vi "LJstreamM write config.vi"(0 "Working Directory":path, 1 "Data File Prefix":string="data", 2 "Scan Rate (Hz)":dbl=100.0 format="%.3f", 3 "Graph History":i32=1000 min=0, 4 "# Channels":i32=4, 5 "filename":string="LJM_Default_Configs.cfg\nLJM_Default_Configs.cfg", 6 "Disable Scaling":bool, 7 "Max File Size (Bytes)":i32=1048576, 9 "Write To File":bool, 10 "Channel Setup":T1={"+Ch"=["0", "1", "2", "3", "4", "5", "6", "7"], "-Ch"=["199", "199", "199", "199", "199", "199", "199", "199"], "Ranges"=[0, 0, 0, 0, 0, 0, 0, 0], "Scaling Equation"=["y=v0", "y=v1", "y=v2", "y=v3", "y=v4", "y=v5", "y=v6", "y=v7"], "Graph?"=[]} {"Ranges" items=["LJ_rgBIP10V", "LJ_rgBIP5V", "LJ_rgUNI5V", "LJ_rgUNI2P5V", "LJ_rgUNI1P25V", "LJ_rgBIP1V", "LJ_rgUNIP625V", "LJ_rgBIPP1V", "LJ_rgBIPP01V"]}, 11 "App Name":string="LJStreamM.cfg", 12 "Interval (ms)":u32=500, 13 "Resolution":u8, 14 "SettlingFactor":u8) -> (15 "error out":errorcluster={"status"=TRUE, "code"=1, "source"="Open/Create/Replace File in NI_LVConfig.lvlib:Load.vi->NI_LVConfig.lvlib:Open Config Data (compatibility).vi->LJstreamM write config.vi<APPEND>\nLJM_Default_Configs.cfg\nLJM_Default_Configs.cfg:\\"})   [LabVIEW 2025]
uses:
  LJstreamM globals.vi
  <vilib>/Utility/config.llb/Write Key (String).vi
  <vilib>/Utility/config.llb/Write Key (U32).vi
  <vilib>/Utility/config.llb/Write Key (Double).vi
  <vilib>/Utility/config.llb/Write Key (I32).vi
  <vilib>/Utility/config.llb/Write Key (Boolean).vi
  <vilib>/Utility/config.llb/NI_LVConfig.lvlib
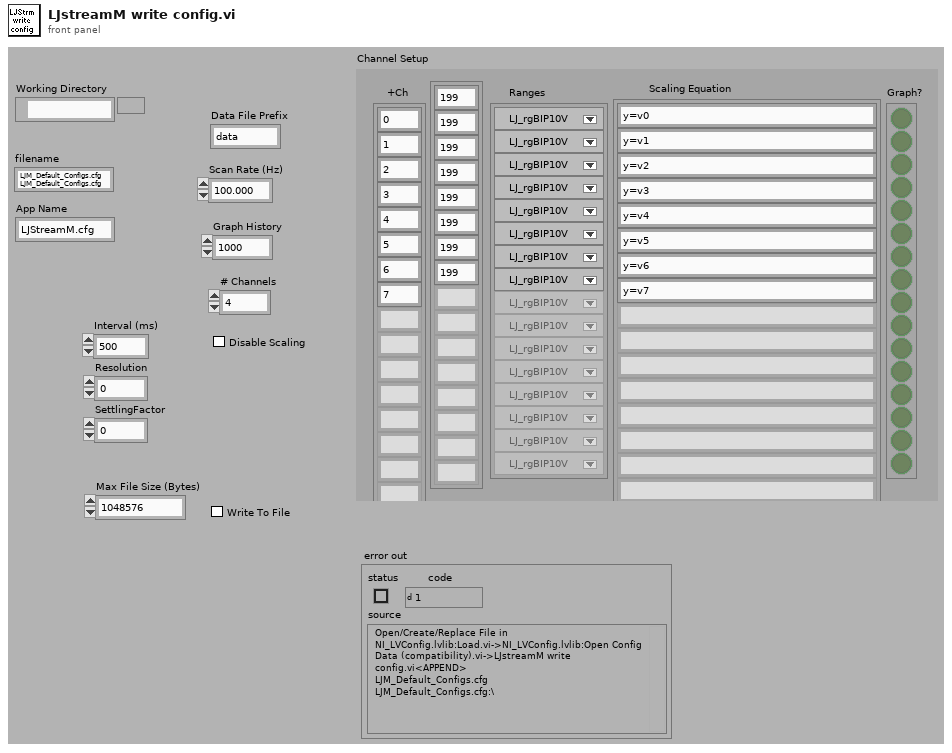
[diagram p1: front panel]
types:
  T1 = cluster{"+Ch":string[], "-Ch":string[], "Ranges":u16[], "Scaling Equation":string[], "Graph?":bool[]}
  T2 = typedef "NI_LVConfig.lvlib/Config Data RefNum.ctl" = refnum<k1>
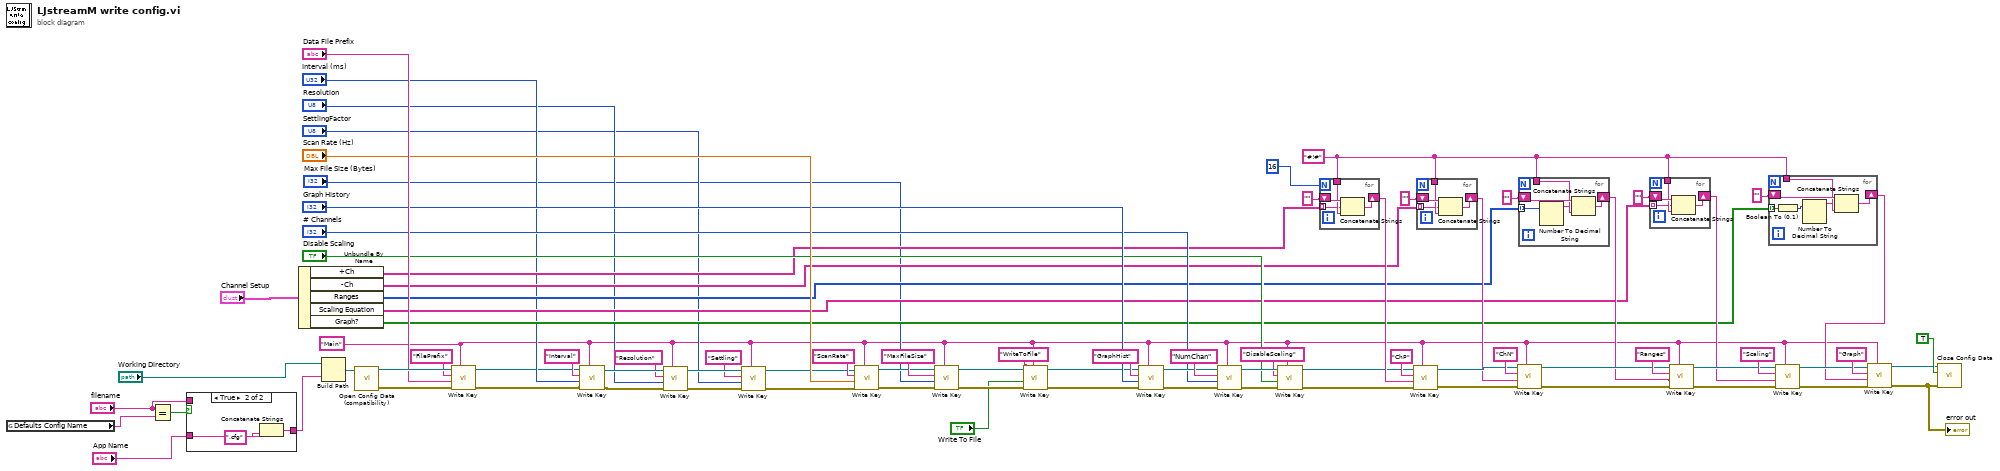
[diagram p0: block diagram]
diagram:
  w47 = "#!#" ("delimiter (Tab)")
  w11 = "Main" ("section")
  n1 = global read "LJstreamM globals.vi" "Defaults Config Name"() -> (w1:string)
  n2 = Equal?(x="filename", y=w1) -> (x = y?=w3:bool)
  n3 = case shown="True" w3 {
    tunnel: [w85 w88] -> w5
    tunnel: "App Name" -> [_ w87]
    tunnel: "filename" -> [w85 _]
    frame False {
    }
    frame True {
      n4 = Concatenate Strings(w87, ".cfg" ("string")) -> (w88:string)
    }
  }
  n5 = Unbundle By Name("Channel Setup") -> ("+Ch"=w32:string[], "-Ch"=w33:string[], "Ranges"=w34:u16[], "Scaling Equation"=w35:string[], "Graph?"=w36:bool[])
  n6 = Build Path(base path="Working Directory", name or relative path=w5) -> (appended path=w84:path)
  n7 = call <vilib>:"Open Config Data (compatibility).vi"("configuration file path"=w84) -> ("error out"=w82:errorcluster, "refnum"=w83:T2)  [unwired: 8 in, 1 out]
  n8 = call-poly <vilib>:"Write Key.vi"("section"=w11, "error in (no error)"=w82, "value"="Data File Prefix", "key"="FilePrefix", "refnum"=w83) -> ("error out"=w20:errorcluster, "refnum out"=w21:T2)  [unwired: 4 in, 1 out]
  n9 = call-poly <vilib>:"Write Key.vi"("section"=w11, "error in (no error)"=w20, "value"="Interval (ms)", "key"="Interval", "refnum"=w21) -> ("error out"=w29:errorcluster, "refnum out"=w28:T2)  [unwired: 4 in, 1 out]
  n10 = call-poly <vilib>:"Write Key.vi"("section"=w11, "error in (no error)"=w29, "value"="Resolution", "key"="Resolution", "refnum"=w28) -> ("error out"=w31:errorcluster, "refnum out"=w30:T2)  [unwired: 4 in, 1 out]
  n11 = call-poly <vilib>:"Write Key.vi"("section"=w11, "error in (no error)"=w31, "value"="SettlingFactor", "key"="Settling", "refnum"=w30) -> ("error out"=w18:errorcluster, "refnum out"=w19:T2)  [unwired: 4 in, 1 out]
  n12 = call-poly <vilib>:"Write Key.vi"("section"=w11, "error in (no error)"=w18, "value"="Scan Rate (Hz)", "key"="ScanRate", "refnum"=w19) -> ("error out"=w15:errorcluster, "refnum out"=w14:T2)  [unwired: 4 in, 1 out]
  n13 = call-poly <vilib>:"Write Key.vi"("section"=w11, "error in (no error)"=w15, "value"="Max File Size (Bytes)", "key"="MaxFileSize", "refnum"=w14) -> ("error out"=w9:errorcluster, "refnum out"=w10:T2)  [unwired: 4 in, 1 out]
  n14 = call-poly <vilib>:"Write Key.vi"("section"=w11, "error in (no error)"=w9, "value"="Write To File", "key"="WriteToFile", "refnum"=w10) -> ("error out"=w7:errorcluster, "refnum out"=w8:T2)  [unwired: 4 in, 1 out]
  n15 = call-poly <vilib>:"Write Key.vi"("section"=w11, "error in (no error)"=w7, "value"="Graph History", "key"="GraphHist", "refnum"=w8) -> ("error out"=w77:errorcluster, "refnum out"=w78:T2)  [unwired: 4 in, 1 out]
  n16 = call-poly <vilib>:"Write Key.vi"("section"=w11, "error in (no error)"=w77, "value"="# Channels", "key"="NumChan", "refnum"=w78) -> ("error out"=w55:errorcluster, "refnum out"=w56:T2)  [unwired: 4 in, 1 out]
  n17 = call-poly <vilib>:"Write Key.vi"("section"=w11, "error in (no error)"=w55, "value"="Disable Scaling", "key"="DisableScaling", "refnum"=w56) -> ("error out"=w54:errorcluster, "refnum out"=w53:T2)  [unwired: 4 in, 1 out]
  n18 = for {
    N: 16 -> [_]
    shift-right: [w91] -> w60
    shift-left: "" -> [w92]
    tunnel: w47 -> [w90]
    tunnel: w32 -> [w89] mode=indexing
    n19 = Concatenate Strings(w92, w89, w90) -> (w91:string)
  }
  n20 = call-poly <vilib>:"Write Key.vi"("section"=w11, "error in (no error)"=w54, "value"=w60, "key"="ChP", "refnum"=w53) -> ("error out"=w72:errorcluster, "refnum out"=w73:T2)  [unwired: 4 in, 1 out]
  n21 = for {
    shift-right: [w95] -> w59
    shift-left: "" -> [w96]
    tunnel: w47 -> [w94]
    tunnel: w33 -> [w93] mode=indexing
    n22 = Concatenate Strings(w96, w93, w94) -> (w95:string)
  }
  n23 = call-poly <vilib>:"Write Key.vi"("section"=w11, "error in (no error)"=w72, "value"=w59, "key"="ChN", "refnum"=w73) -> ("error out"=w71:errorcluster, "refnum out"=w70:T2)  [unwired: 4 in, 1 out]
  n24 = for {
    shift-right: [w100] -> w58
    shift-left: "" -> [w101]
    tunnel: w47 -> [w99]
    tunnel: w34 -> [w98] mode=indexing
    n25 = Number To Decimal String(number=w98) -> (decimal integer string=w97:string)  [unwired: 1 in]
    n26 = Concatenate Strings(w101, w97, w99) -> (w100:string)
  }
  n27 = for {
    shift-right: [w104] -> w57
    shift-left: "" -> [w105]
    tunnel: w47 -> [w103]
    tunnel: w35 -> [w102] mode=indexing
    n28 = Concatenate Strings(w105, w102, w103) -> (w104:string)
  }
  n29 = call-poly <vilib>:"Write Key.vi"("section"=w11, "error in (no error)"=w71, "value"=w58, "key"="Ranges", "refnum"=w70) -> ("error out"=w68:errorcluster, "refnum out"=w67:T2)  [unwired: 4 in, 1 out]
  n30 = for {
    shift-right: [w110] -> w46
    shift-left: "" -> [w111]
    tunnel: w47 -> [w109]
    tunnel: w36 -> [w106] mode=indexing
    n31 = Boolean To (0,1)(Boolean=w106) -> (0, 1=w107:i16)
    n32 = Number To Decimal String(number=w107) -> (decimal integer string=w108:string)  [unwired: 1 in]
    n33 = Concatenate Strings(w111, w108, w109) -> (w110:string)
  }
  n34 = call-poly <vilib>:"Write Key.vi"("section"=w11, "error in (no error)"=w68, "value"=w57, "key"="Scaling", "refnum"=w67) -> ("error out"=w49:errorcluster, "refnum out"=w48:T2)  [unwired: 4 in, 1 out]
  n35 = call-poly <vilib>:"Write Key.vi"("section"=w11, "error in (no error)"=w49, "value"=w46, "key"="Graph", "refnum"=w48) -> ("error out"=w37:errorcluster, "refnum out"=w45:T2)  [unwired: 4 in, 1 out]
  "error out" <- w37
  n36 = call <vilib>:"Close Config Data.vi"("error in (no error)"=w37, "write file if changed (T)"=TRUE ("write configuration file? (F)"), "refnum"=w45) -> ()  [unwired: 7 in, 2 out]
